vi "Get_AttributeValue.vi"(8 "error in (no error)":errorcluster, 10 "AttributesName":string, 11 "Node Reg in":refnum<k20>) -> (0 "error out":errorcluster, 2 "AttributesValue":string, 3 "Node Reg out":refnum<k20>)   [LabVIEW 2010, in "Pansino_XML_Read.lvlib"]
uses:
  <vilib>/xml/Close Reference(Node).vi
  <vilib>/xml/Close Reference(NNMap).vi
  Pansino_XML_Read.lvlib
  C:/Program Files (x86)/National Instruments/LabVIEW 2010/resource/objmgr/DOMUserDefRef.rc
  <vilib>/xml/NI_XML.lvlib
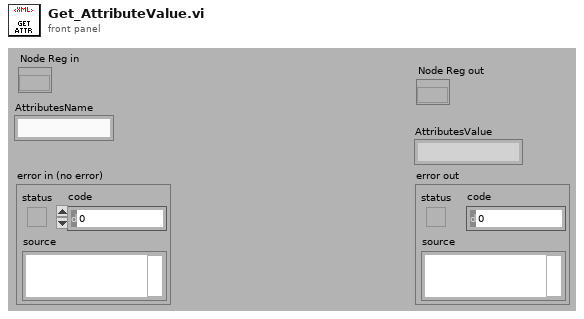
[diagram p1: front panel]
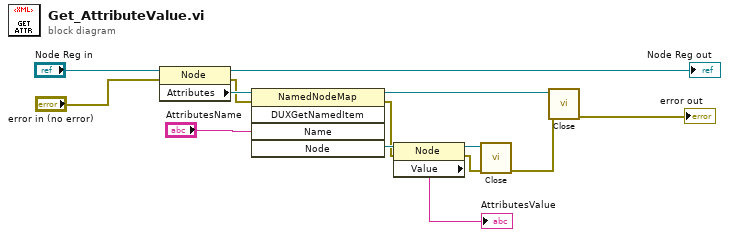
[diagram p0: block diagram]
diagram:
  n1 = property class="Node"(reference="Node Reg in", error in="error in (no error)") -> (reference out=→"Node Reg out":refnum<k20>, error out=w3:errorcluster, "Attributes"=w6:refnum<k20>)
  n2 = invoke class="NamedNodeMap" method="DUXGetNamedItem"(reference=w6, error in=w3, "Name"="AttributesName") -> (reference out=w11:refnum<k20>, error out=w4:errorcluster, "Node"=w8:refnum<k20>)  [unwired: 2 in, 2 out]
  n3 = property class="Node"(reference=w8, error in=w4) -> (reference out=w10:refnum<k20>, error out=w13:errorcluster, "Value"=→"AttributesValue":string)
  n4 = call-poly <vilib>:"Close.vi"("error in (no error)"=w13, "node"=w10) -> ("error out"=w1:errorcluster)  [unwired: 7 out]
  n5 = call-poly <vilib>:"Close.vi"("error in (no error)"=w1, "named node map"=w11) -> ("error out"=→"error out":errorcluster)  [unwired: 7 out]
